vi "UTILITY Extract Plot Data.vi"(7 "Plot Array in":dbl[][](array[numeric]), 8 "Error In":errorcluster, 9 "Save Data":string[](array[string]), 11 "Axis":string) -> (0 "Error Out":errorcluster, 3 "Plot Array out":dbl[](array[numeric]))   [LabVIEW 2019]
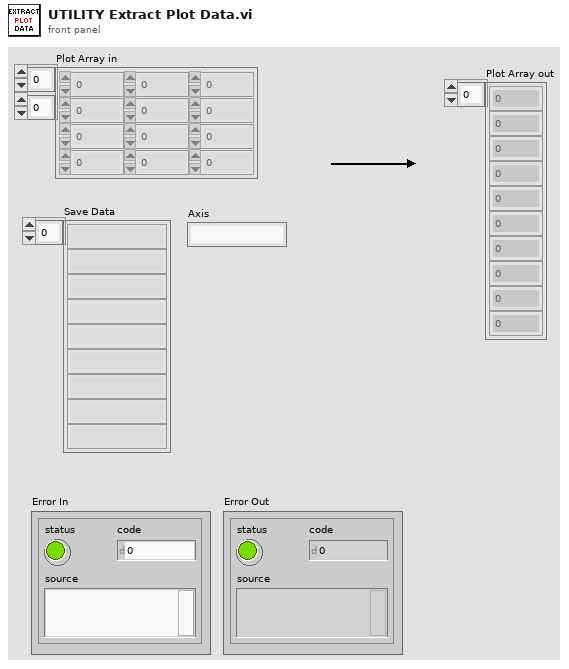
[diagram p1: front panel]
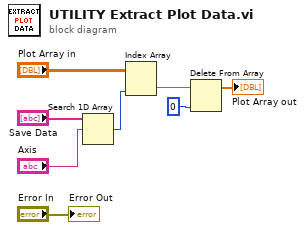
[diagram p0: block diagram]
diagram:
  n1 = Search 1D Array(1D array="Save Data", element="Axis") -> (index of element=w6:i32)  [unwired: 1 in]
  n2 = Index Array(array="Plot Array in", index (col)=w6) -> (element=w5:dbl[])  [unwired: 1 in]
  n3 = Delete From Array(array=w5, index=0) -> (array with subset deleted=→"Plot Array out":dbl[])  [unwired: 1 in, 1 out]
  "Error Out" <- "Error In"
